vi "stage-controller.vi"() -> ()   [LabVIEW 2014]
uses:
  Stage SubVis/Move stage command - Global - SubVI.ctl
  Stage SubVis/user event out globals - SubVI.vi
  Stage SubVis/field-raster-globals.vi
  lib/Madlib/Madlib.lvlib
panel:
  in  "Current Z 2":ext(slide)=5.551115123125783e-17 scale=-1.0..1.0 scale format="%_1f"
  out "Current (X,Y)":cluster{ext[], ext[]}[](graph)=[{[101.064], [100.915]}, {[67.376, 134.75199999999998], [134.55333333333334, 134.55333333333334]}, {[67.376, 134.75199999999998], [67.27666666666667, 67.27666666666667]}]
  in  "Field Number":u32(slide)=1 min=1 max=16 step=1 scale=1.0..16.0
  in  "Field Size":enum16{"0", "1", "4", "9", "16"}(ring)=enum."9"
  in  "x-":bool
  in  "y+":bool
  in  "y-":bool
  in  "x+":bool
  out "Current Z (um)":ext
  out "Current X (um)":ext
  out "Current Y (um)":ext
  in  "Current Z":dbl(slide) min=0.0 step=0.5 scale=0.0..202.234 scale format="%#_4g"
  out "At limit 3":bool
  out "At limit 2":bool
  out "At limit":bool
  in  "x,y step (um)":ext=10.0 format="%_5g"
  in  "z step (um)":ext(slide)=0.1 scale=0.05..2.0 scale format="%#_2g"
  in  "z-":bool
  in  "z+":bool
  in  "Reset stage to center\n         (x, y, and z)":bool
  in  "STOP":bool
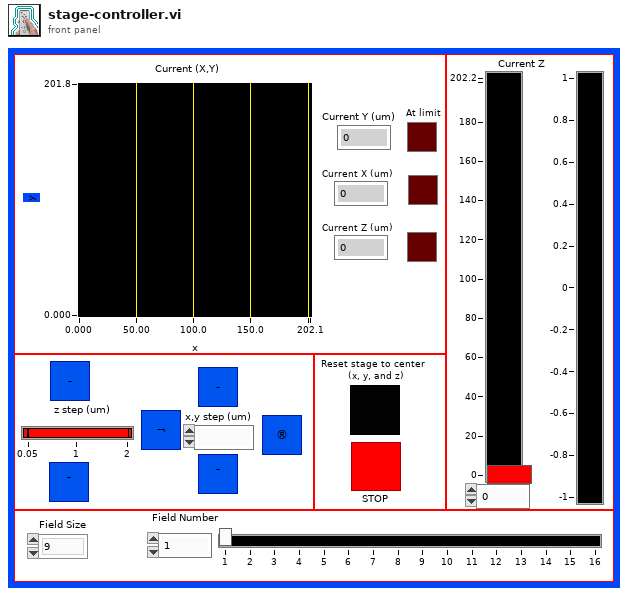
[diagram p1: front panel]
types:
  T1 = cluster{"X Command":dbl, "Y Command":dbl, "Z Command":dbl, "X Position":dbl, "Y Position":dbl, "Z Position":dbl, "X Calibration":dbl, "Y Calibration":dbl, "Z Calibration":dbl}
  T2 = typedef "Move stage command - Global - SubVI.ctl" = cluster{"dx (um) (0 -> ignore)":ext, "dy (um) (0 -> ignore)":ext, "dz (um) (0 -> ignore)":ext, "Re-center x,y":bool, "Re-center z":bool, "x (um) (-1 -> ignore)":dbl, "y (um) (-1 -> ignore)":dbl, "z (um) (-1 -> ignore)":dbl}
  T3 = typedef "small z increment.ctl" = dbl
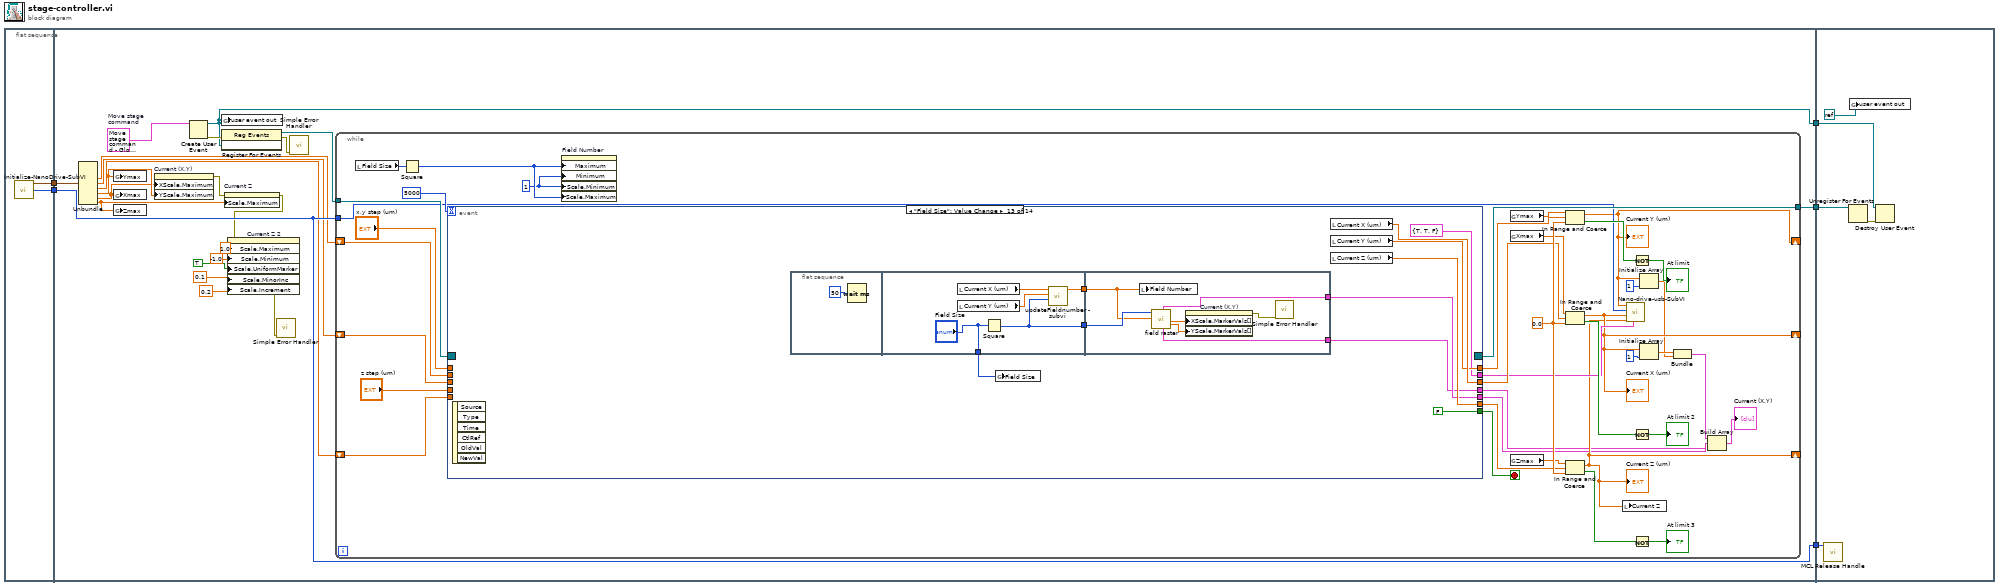
[diagram p0: block diagram]
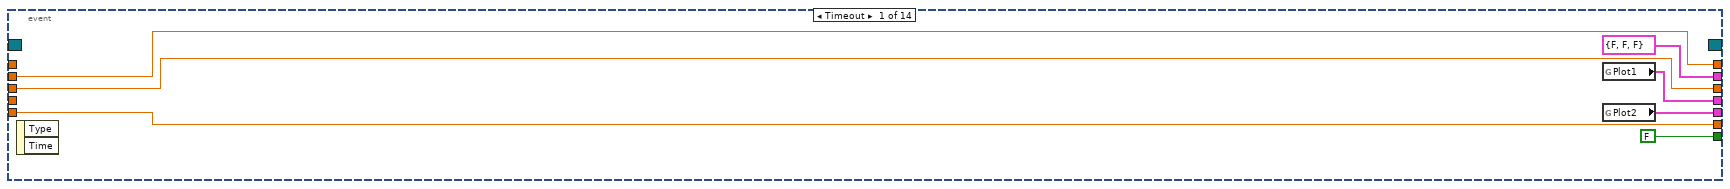
[diagram p2: hidden frame]
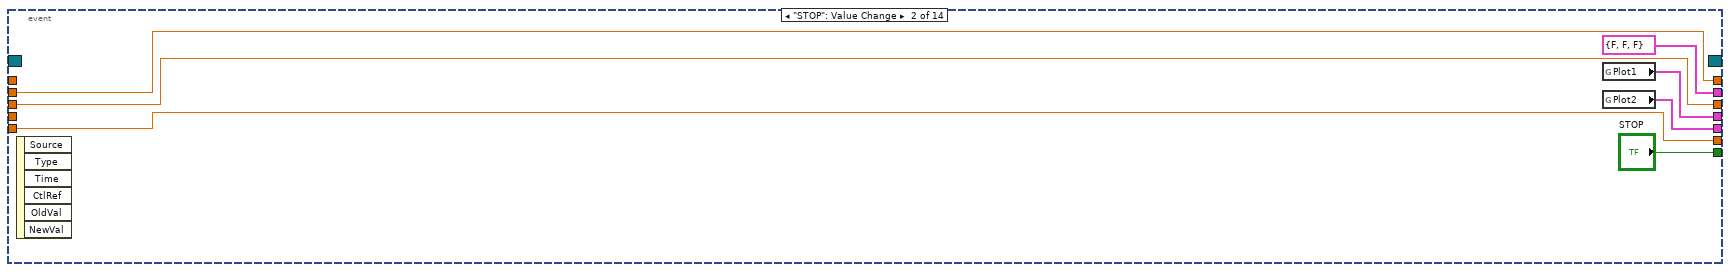
[diagram p3: hidden frame]
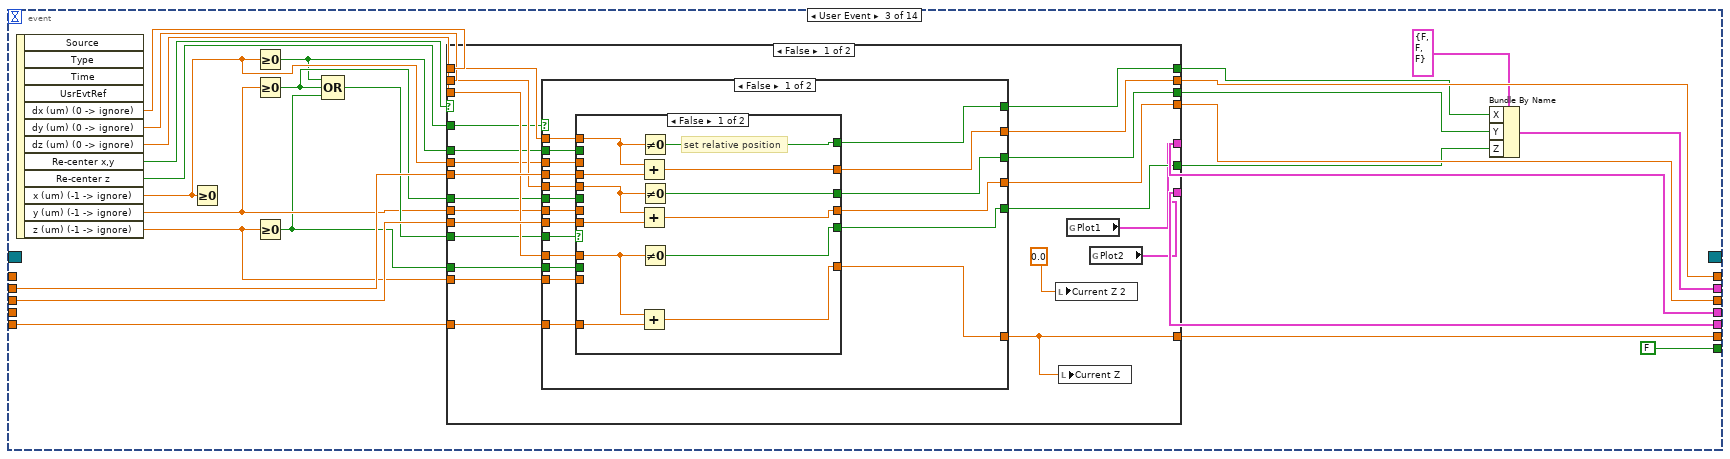
[diagram p4: hidden frame]
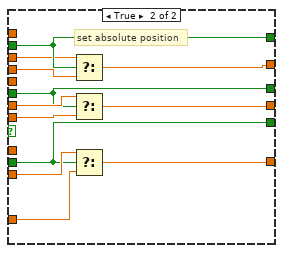
[diagram p5: hidden frame]
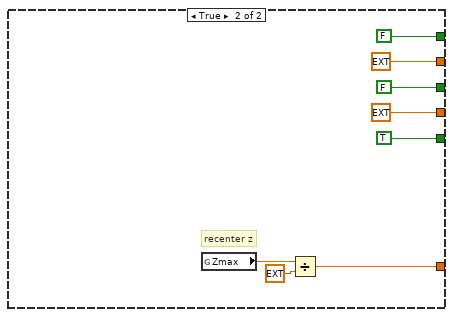
[diagram p6: hidden frame]
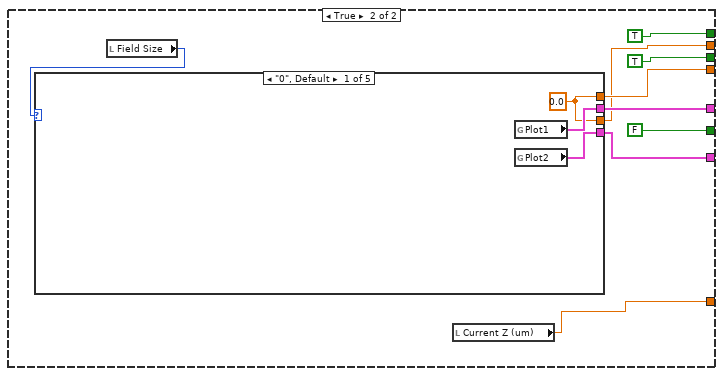
[diagram p7: hidden frame]
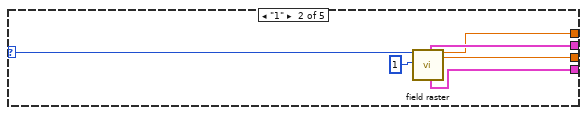
[diagram p8: hidden frame]
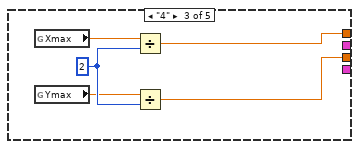
[diagram p9: hidden frame]
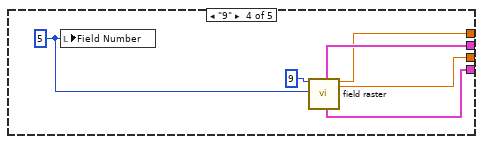
[diagram p10: hidden frame]
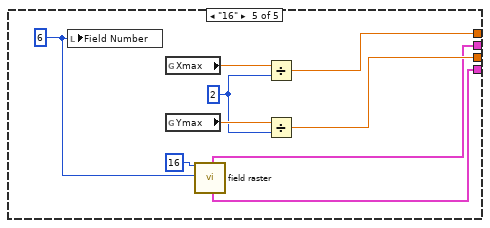
[diagram p11: hidden frame]
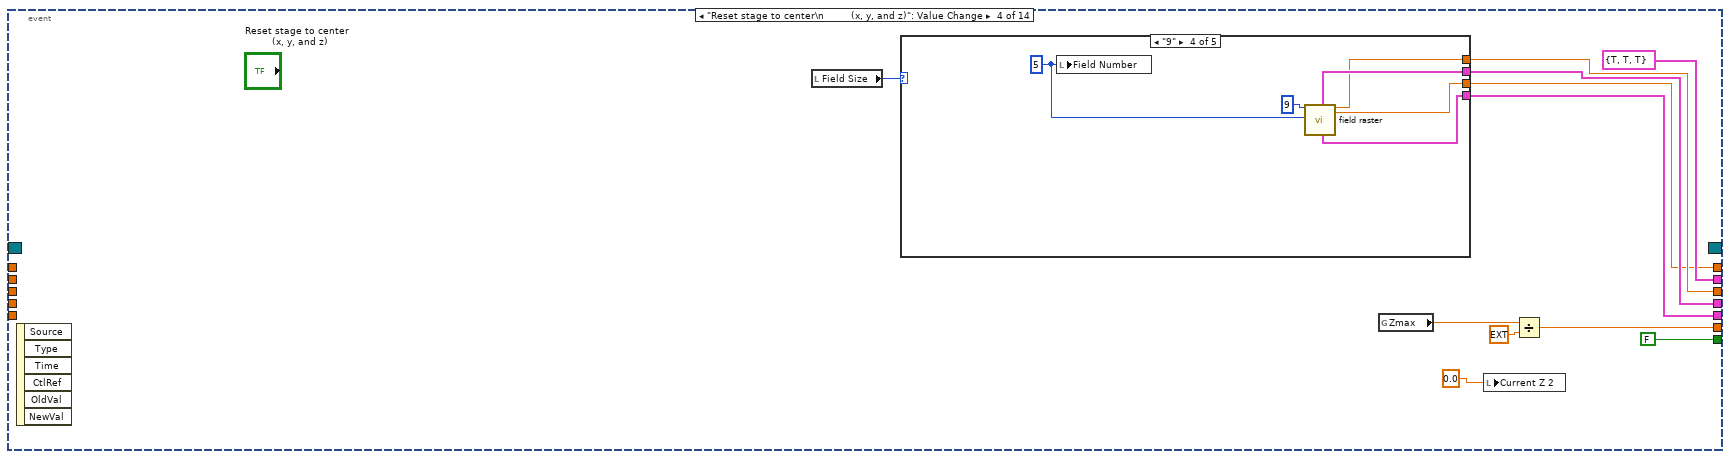
[diagram p12: hidden frame]
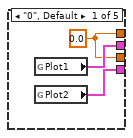
[diagram p13: hidden frame]
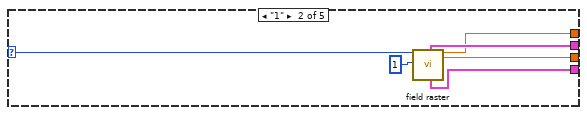
[diagram p14: hidden frame]
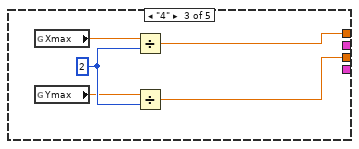
[diagram p15: hidden frame]
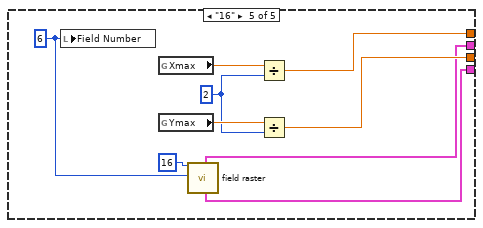
[diagram p16: hidden frame]
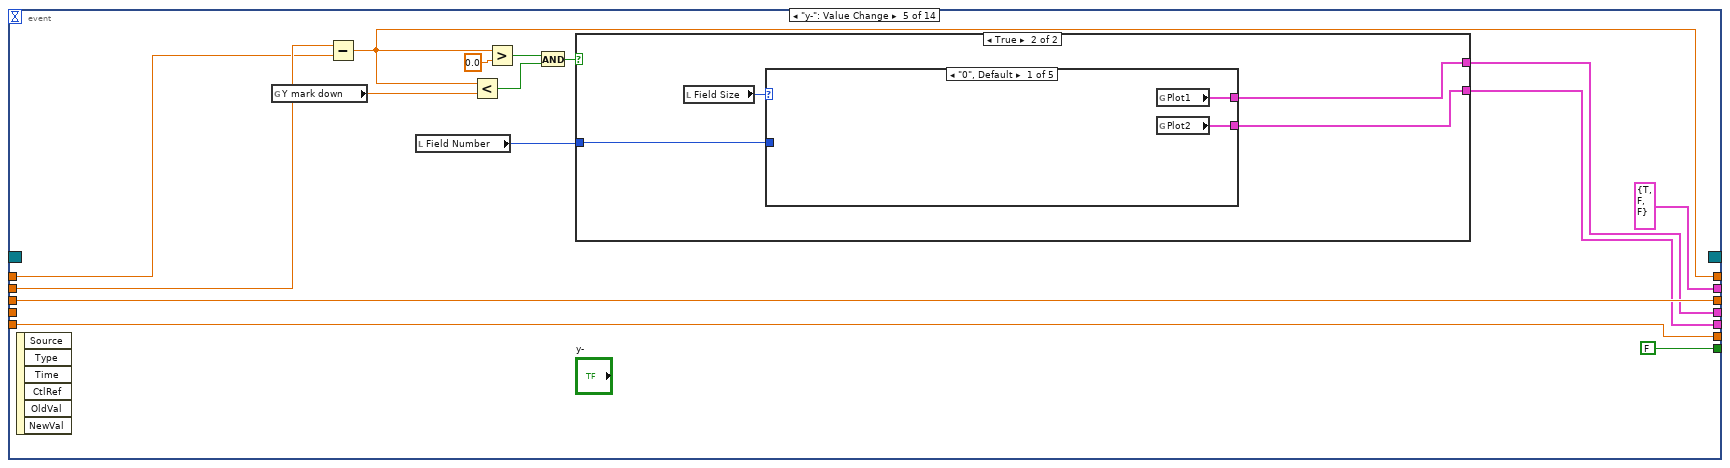
[diagram p17: hidden frame]
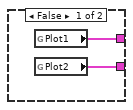
[diagram p18: hidden frame]
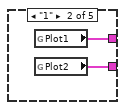
[diagram p19: hidden frame]
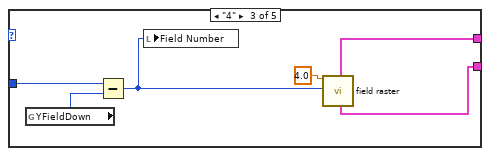
[diagram p20: hidden frame]
diagram:
  n1 = flat-sequence {
    tunnel: [w7] -> w5
    tunnel: [w6] -> w2
    tunnel: w5 -> [w29]
    tunnel: [w24] -> w4
    tunnel: [w23] -> w3
    tunnel: w2 -> [w22]
    tunnel: [w22] -> w1
    tunnel: w4 -> [w518]
    tunnel: w3 -> [w517]
    tunnel: w1 -> [w515]
    frame #0 {
      n2 = call "Initialize-NanoDrive-SubVI.vi"() -> ("Output Pos Info"=w7:T1, "Handle"=w6:i32)  [unwired: 1 in, 1 out]
    }
    frame #1 {
      w28 = T2 {"dx (um) (0 -> ignore)"=0.0, "dy (um) (0 -> ignore)"=0.0, "dz (um) (0 -> ignore)"=0.0, "Re-center x,y"=FALSE, "Re-center z"=FALSE, "x (um) (-1 -> ignore)"=-1.0, "y (um) (-1 -> ignore)"=-1.0, "z (um) (-1 -> ignore)"=-1.0}  # Move stage command
      n3 = Unbundle(w29) -> ("X Position"=w21:dbl, "Y Position"=w20:dbl, "Z Position"=w19:dbl, "X Calibration"=w17:dbl, "Y Calibration"=w16:dbl, "Z Calibration"=w15:dbl)  [unwired: 3 out]
      n4 = global write "field-raster-globals.vi" "Ymax"(w17) -> ()
      n5 = global write "field-raster-globals.vi" "Xmax"(w16) -> ()
      n6 = global write "field-raster-globals.vi" "Zmax"(w15) -> ()
      n7 = property on="Current (X,Y)" class="XYGraph (strict)"("XScale.Maximum"=w16, "YScale.Maximum"=w17) -> (error out=w18:errorcluster)  [unwired: 2 in, 1 out]
      n8 = Create User Event(user event datatype=w28) -> (user event=w23:refnum<user-event>, error out=w26:errorcluster)  [unwired: 1 in]
      n9 = global write "user event out globals - SubVI.vi" "user event out"(w23) -> ()
      n10 = register-events(error in=w26, w23) -> (reference out=w25:refnum<event-registration>, error out=w27:errorcluster)  [unwired: 1 in]
      n11 = property on="Current Z" class="Slide (strict)"(error in=w18, "Scale.Maximum"=w15) -> (error out=w14:errorcluster)  [unwired: 1 in, 1 out]
      n12 = property on="Current Z 2" class="Slide (strict)"(error in=w14, "Scale.Maximum"=1.0 ("Scale.Range:Maximum"), "Scale.Minimum"=-1.0 ("Scale.Range:Minimum"), "Scale.UniformMarker"=TRUE, "Scale.MinorInc"=0.1 ("Scale.Range:Minor Increment"), "Scale.Increment"=0.2 ("Scale.Range:Increment")) -> (error out=w13:errorcluster)  [unwired: 1 in, 1 out]
      n13 = call <vilib>:"Simple Error Handler.vi"("error in (no error)"=w13) -> ()  [unwired: 4 in, 5 out]
      n14 = call <vilib>:"Simple Error Handler.vi"("error in (no error)"=w27) -> ()  [unwired: 1 in, 8 out]
      n15 = while {
        tunnel: w25 -> [w65]
        tunnel: [w64] -> w24
        tunnel: w22 -> [w49]
        shift-right: [w45] -> _
        shift-left: w21 -> [w48]
        shift-right: [w44] -> _
        shift-left: w20 -> [w47]
        shift-right: [w40] -> _
        shift-left: w19 -> [w46]
        stop <- w66 stop-if-true
        w37 = 1
        w63 = 0.0
        n16 = local read "Field Size"() -> (w39:enum16{"0", "1", "4", "9", "16"})
        n17 = Square(x=w39) -> (x^2=w38:u16)
        n18 = event shown="[12] \"Field Size\": Value Change" {
          selector: w65 -> [_ _ _ _ _ _ _ _ _ _ _ _ _ _]
          dyn-events: [_ _ _ _ _ _ _ _ _ _ _ _ _ _] -> w64
          timeout: 5000 -> [_ _ _ _ _ _ _ _ _ _ _ _ _ _]
          tunnel: [FALSE ("Stop") "STOP" FALSE ("Stop") FALSE ("Stop") FALSE ("Stop") FALSE ("Stop") FALSE ("Stop") FALSE ("Stop") FALSE ("Stop") FALSE ("Stop") FALSE ("Stop") FALSE ("Stop") FALSE FALSE] -> w66
          tunnel: w48 -> [w73 w80 w107 _ w270 w310 w317 w328 w347 w358 w405 w445 _ _]
          tunnel: w47 -> [w72 w79 w106 _ w273 w305 w316 w327 w346 w362 w402 w449 _ _]
          tunnel: w46 -> [w71 w78 w105 _ w272 w307 _ w325 w343 w363 w406 w448 _ _]
          tunnel: [w73 w80 w102 w222 w261 w310 w317 w328 w347 w358 w405 w437 w487 w508] -> w62
          tunnel: [w72 w79 w103 w223 w273 w305 w316 w327 w346 w351 w394 w449 w488 w507] -> w61
          tunnel: [w71 w78 w104 w228 w272 w309 "Current Z" w324 w349 w363 w406 w448 w485 w503] -> w60
          tunnel: [cluster{"X":bool, "Y":bool, "Z":bool} {"X"=FALSE, "Y"=FALSE, "Z"=FALSE} ("Set this axis?") cluster{"X":bool, "Y":bool, "Z":bool} {"X"=FALSE, "Y"=FALSE, "Z"=FALSE} ("Set this axis?") w95 cluster{"X":bool, "Y":bool, "Z":bool} {"X"=TRUE, "Y"=TRUE, "Z"=TRUE} ("Set this axis?") cluster{"X":bool, "Y":bool, "Z":bool} {"X"=TRUE, "Y"=FALSE, "Z"=FALSE} ("Set this axis?") cluster{"X":bool, "Y":bool, "Z":bool} {"X"=FALSE, "Y"=FALSE, "Z"=TRUE} ("Set this axis?") cluster{"X":bool, "Y":bool, "Z":bool} {"X"=FALSE, "Y"=FALSE, "Z"=TRUE} ("Set this axis?") cluster{"X":bool, "Y":bool, "Z":bool} {"X"=FALSE, "Y"=FALSE, "Z"=TRUE} ("Set this axis?") cluster{"X":bool, "Y":bool, "Z":bool} {"X"=FALSE, "Y"=FALSE, "Z"=TRUE} ("Set this axis?") cluster{"X":bool, "Y":bool, "Z":bool} {"X"=FALSE, "Y"=TRUE, "Z"=FALSE} ("Set this axis?") cluster{"X":bool, "Y":bool, "Z":bool} {"X"=FALSE, "Y"=TRUE, "Z"=FALSE} ("Set this axis?") cluster{"X":bool, "Y":bool, "Z":bool} {"X"=TRUE, "Y"=FALSE, "Z"=FALSE} ("Set this axis?") cluster{"X":bool, "Y":bool, "Z":bool} {"X"=TRUE, "Y"=TRUE, "Z"=FALSE} ("Set this axis?") cluster{"X":bool, "Y":bool, "Z":bool} {"X"=TRUE, "Y"=TRUE, "Z"=FALSE} ("Set this axis?")] -> w50
          tunnel: "x,y step (um)" -> [_ _ _ _ w269 _ _ _ _ w361 w403 w446 _ _]
          tunnel: "z step (um)" -> [_ _ _ _ _ w306 _ _ w344 _ _ _ _ _]
          tunnel: [w68 w75 w82 w225 w266 w304 w313 w331 w342 w356 w399 w442 w483 w509] -> w35
          tunnel: [w69 w76 w83 w226 w267 w303 w314 w330 w341 w357 w400 w443 w482 w510] -> w34
          event Timeout {
            n19 = event-data() -> ()  [unwired: 3 out]
            n20 = global read "field-raster-globals.vi" "Plot1"() -> (w69:cluster{dbl[], dbl[]})
            n21 = global read "field-raster-globals.vi" "Plot2"() -> (w68:cluster{dbl[], dbl[]})
          }
          event "STOP": Value Change {
            n22 = event-data() -> ()  [unwired: 7 out]
            n23 = global read "field-raster-globals.vi" "Plot1"() -> (w76:cluster{dbl[], dbl[]})
            n24 = global read "field-raster-globals.vi" "Plot2"() -> (w75:cluster{dbl[], dbl[]})
          }
          event User Event {
            n25 = event-data() -> ("dx (um) (0 -> ignore)"=w100:ext, "dy (um) (0 -> ignore)"=w99:ext, "dz (um) (0 -> ignore)"=w98:ext, "Re-center x,y"=w97:bool, "Re-center z"=w91:bool, "x (um) (-1 -> ignore)"=w87:dbl, "y (um) (-1 -> ignore)"=w88:dbl, "z (um) (-1 -> ignore)"=w89:dbl)  [unwired: 5 out]
            n26 = Greater Or Equal To 0?(x=w87) -> ()  [unwired: 1 out]
            n27 = Greater Or Equal To 0?(x=w87) -> (x >= 0?=w84:bool)
            n28 = Greater Or Equal To 0?(x=w88) -> (x >= 0?=w85:bool)
            n29 = Greater Or Equal To 0?(x=w89) -> (x >= 0?=w86:bool)
            n30 = Compound Arithmetic op=OR(w84, w85, w86) -> (w90:bool)
            n31 = case shown="False" w97 {
              tunnel: w107 -> [w130 _]
              tunnel: w106 -> [w129 _]
              tunnel: w105 -> [w128 _]
              tunnel: [w111 w183] -> w104
              tunnel: [w127 w185] -> w103
              tunnel: [w126 w184] -> w102
              tunnel: w100 -> [w125 _]
              tunnel: w99 -> [w124 _]
              tunnel: w98 -> [w123 _]
              tunnel: [w122 FALSE] -> w94
              tunnel: [w121 TRUE] -> w93
              tunnel: [w120 TRUE] -> w92
              tunnel: w91 -> [w119 _]
              tunnel: w90 -> [w118 _]
              tunnel: w89 -> [w117 _]
              tunnel: w88 -> [w116 _]
              tunnel: w87 -> [w115 _]
              tunnel: w86 -> [w114 _]
              tunnel: w85 -> [w113 _]
              tunnel: w84 -> [w112 _]
              tunnel: [w109 w187] -> w83
              tunnel: [w108 w186] -> w82
              frame False {
                n32 = case shown="False" w119 {
                  tunnel: w130 -> [w149 _]
                  tunnel: w129 -> [w148 _]
                  tunnel: w128 -> [w147 _]
                  tunnel: [w146 w180] -> w111
                  tunnel: [w145 ext 0.0] -> w127
                  tunnel: [w144 ext 0.0] -> w126
                  tunnel: w125 -> [w143 _]
                  tunnel: w124 -> [w142 _]
                  tunnel: w123 -> [w141 _]
                  tunnel: [w140 TRUE] -> w122
                  tunnel: [w139 FALSE] -> w121
                  tunnel: [w138 FALSE] -> w120
                  tunnel: w118 -> [w137 _]
                  tunnel: w117 -> [w136 _]
                  tunnel: w116 -> [w135 _]
                  tunnel: w115 -> [w134 _]
                  tunnel: w114 -> [w133 _]
                  tunnel: w113 -> [w132 _]
                  tunnel: w112 -> [w131 _]
                  frame False {
                    n33 = case shown="False" w137 {
                      tunnel: w149 -> [w161 w169]
                      tunnel: w148 -> [w160 w166]
                      tunnel: w147 -> [w159 w163]
                      tunnel: [w158 w165] -> w146
                      tunnel: [w157 w168] -> w145
                      tunnel: [w156 w172] -> w144
                      tunnel: w143 -> [w155 _]
                      tunnel: w142 -> [w154 _]
                      tunnel: w141 -> [w153 _]
                      tunnel: [w152 w162] -> w140
                      tunnel: [w151 w167] -> w139
                      tunnel: [w150 w171] -> w138
                      tunnel: w136 -> [_ w164]
                      tunnel: w135 -> [_ w173]
                      tunnel: w134 -> [_ w170]
                      tunnel: w133 -> [_ w162]
                      tunnel: w132 -> [_ w167]
                      tunnel: w131 -> [_ w171]
                      frame False {
                        # "set relative position"
                        n34 = Add(x=w155, y=w161) -> (x+y=w156:ext)
                        n35 = Add(x=w154, y=w160) -> (x+y=w157:ext)
                        n36 = Add(x=w153, y=w159) -> (x+y=w158:ext)
                        n37 = Not Equal To 0?(x=w155) -> (x != 0?=w150:bool)
                        n38 = Not Equal To 0?(x=w154) -> (x != 0?=w151:bool)
                        n39 = Not Equal To 0?(x=w153) -> (x != 0?=w152:bool)
                      }
                      frame True {
                        # "set absolute position"
                        n40 = Select(t=w170, s=w171, f=w169) -> (s? t:f=w172:ext)
                        n41 = Select(t=w173, s=w167, f=w166) -> (s? t:f=w168:ext)
                        n42 = Select(t=w164, s=w162, f=w163) -> (s? t:f=w165:ext)
                      }
                    }
                  }
                  frame True {
                    # "recenter z"
                    n43 = global read "field-raster-globals.vi" "Zmax"() -> (w174:dbl)
                    n44 = Divide(x=w174, y=ext 2.0) -> (x/y=w180:ext)
                  }
                }
                n45 = local write "Current Z 2"(0.0) -> ()
                n46 = local write "Current Z"(w111) -> ()
                n47 = global read "field-raster-globals.vi" "Plot1"() -> (w109:cluster{dbl[], dbl[]})
                n48 = global read "field-raster-globals.vi" "Plot2"() -> (w108:cluster{dbl[], dbl[]})
              }
              frame True {
                n49 = local read "Field Size"() -> (w182:enum16{"0", "1", "4", "9", "16"})
                n50 = case shown="\"0\", Default" w182 {
                  selector: w182 -> [_ w197 _ _ _]
                  tunnel: [w192 w199 _ w208 w214] -> w187
                  tunnel: [w193 w198 _ w207 w213] -> w186
                  tunnel: [w191 w195 w204 w206 w217] -> w184
                  tunnel: [w191 w194 w203 w205 w216] -> w185
                  frame "0", Default {
                    w191 = 0.0
                    n51 = global read "field-raster-globals.vi" "Plot1"() -> (w192:cluster{dbl[], dbl[]})
                    n52 = global read "field-raster-globals.vi" "Plot2"() -> (w193:cluster{dbl[], dbl[]})
                  }
                  frame "1" {
                    n53 = call "field raster.vi"("field size"=w197, "field number"=1) -> ("Plot1"=w199:cluster{dbl[], dbl[]}, "Plot2"=w198:cluster{dbl[], dbl[]}, "current X"=w194:dbl, "current Y"=w195:dbl)  [unwired: 12 in, 2 out]
                  }
                  frame "4" {
                    w202 = 2
                    n54 = global read "field-raster-globals.vi" "Xmax"() -> (w201:dbl)
                    n55 = global read "field-raster-globals.vi" "Ymax"() -> (w200:dbl)
                    n56 = Divide(x=w201, y=w202) -> (x/y=w203:dbl)
                    n57 = Divide(x=w200, y=w202) -> (x/y=w204:dbl)
                  }
                  frame "9" {
                    w209 = 5
                    n58 = local write "Field Number"(w209) -> ()
                    n59 = call "field raster.vi"("field size"=9, "field number"=w209) -> ("Plot1"=w208:cluster{dbl[], dbl[]}, "Plot2"=w207:cluster{dbl[], dbl[]}, "current X"=w205:dbl, "current Y"=w206:dbl)  [unwired: 12 in, 2 out]
                  }
                  frame "16" {
                    w212 = 2
                    w211 = 6
                    n60 = local write "Field Number"(w211) -> ()
                    n61 = global read "field-raster-globals.vi" "Xmax"() -> (w218:dbl)
                    n62 = global read "field-raster-globals.vi" "Ymax"() -> (w219:dbl)
                    n63 = call "field raster.vi"("field size"=16, "field number"=w211) -> ("Plot1"=w214:cluster{dbl[], dbl[]}, "Plot2"=w213:cluster{dbl[], dbl[]})  [unwired: 12 in, 4 out]
                    n64 = Divide(x=w218, y=w212) -> (x/y=w216:dbl)
                    n65 = Divide(x=w219, y=w212) -> (x/y=w217:dbl)
                  }
                }
                n66 = local read "Current Z (um)"() -> (w183:ext)
              }
            }
            n67 = Bundle By Name(cluster=cluster{"X":bool, "Y":bool, "Z":bool} {"X"=FALSE, "Y"=FALSE, "Z"=FALSE} ("Set this axis?"), "X"=w92, "Y"=w93, "Z"=w94) -> (w95:cluster{"X":bool, "Y":bool, "Z":bool})
          }
          event "Reset stage to center\n         (x, y, and z)": Value Change {
            n68 = event-data() -> ()  [unwired: 7 out]
            n69 = local read "Field Size"() -> (w224:enum16{"0", "1", "4", "9", "16"})
            n70 = case shown="\"9\"" w224 {
              selector: w224 -> [_ w237 _ _ _]
              tunnel: [w232 w239 _ w248 w254] -> w226
              tunnel: [w233 w238 _ w247 w253] -> w225
              tunnel: [w231 w235 w244 w246 w257] -> w222
              tunnel: [w231 w234 w243 w245 w256] -> w223
              frame "0", Default {
                w231 = 0.0
                n71 = global read "field-raster-globals.vi" "Plot1"() -> (w232:cluster{dbl[], dbl[]})
                n72 = global read "field-raster-globals.vi" "Plot2"() -> (w233:cluster{dbl[], dbl[]})
              }
              frame "1" {
                n73 = call "field raster.vi"("field size"=w237, "field number"=1) -> ("Plot1"=w239:cluster{dbl[], dbl[]}, "Plot2"=w238:cluster{dbl[], dbl[]}, "current X"=w234:dbl, "current Y"=w235:dbl)  [unwired: 12 in, 2 out]
              }
              frame "4" {
                w242 = 2
                n74 = global read "field-raster-globals.vi" "Xmax"() -> (w241:dbl)
                n75 = global read "field-raster-globals.vi" "Ymax"() -> (w240:dbl)
                n76 = Divide(x=w241, y=w242) -> (x/y=w243:dbl)
                n77 = Divide(x=w240, y=w242) -> (x/y=w244:dbl)
              }
              frame "9" {
                w249 = 5
                n78 = local write "Field Number"(w249) -> ()
                n79 = call "field raster.vi"("field size"=9, "field number"=w249) -> ("Plot1"=w248:cluster{dbl[], dbl[]}, "Plot2"=w247:cluster{dbl[], dbl[]}, "current X"=w245:dbl, "current Y"=w246:dbl)  [unwired: 12 in, 2 out]
              }
              frame "16" {
                w252 = 2
                w251 = 6
                n80 = local write "Field Number"(w251) -> ()
                n81 = global read "field-raster-globals.vi" "Xmax"() -> (w258:dbl)
                n82 = global read "field-raster-globals.vi" "Ymax"() -> (w259:dbl)
                n83 = call "field raster.vi"("field size"=16, "field number"=w251) -> ("Plot1"=w254:cluster{dbl[], dbl[]}, "Plot2"=w253:cluster{dbl[], dbl[]})  [unwired: 12 in, 4 out]
                n84 = Divide(x=w258, y=w252) -> (x/y=w256:dbl)
                n85 = Divide(x=w259, y=w252) -> (x/y=w257:dbl)
              }
            }
            n86 = global read "field-raster-globals.vi" "Zmax"() -> (w221:dbl)
            n87 = local write "Current Z 2"(0.0) -> ()
            n88 = Divide(x=w221, y=ext 2.0) -> (x/y=w228:ext)
          }
          event "y-": Value Change {
            n89 = event-data() -> ()  [unwired: 7 out]
            n90 = global read "field-raster-globals.vi" "Y mark down"() -> (w268:dbl)
            n91 = Subtract(x=w270, y=w269) -> (x-y=w261:ext)
            n92 = local read "Field Number"() -> (w260:u32)
            n93 = Less?(x=w261, y=w268) -> (x < y?=w265:bool)
            n94 = Greater?(x=w261, y=0.0) -> (0:w263:bool)
            n95 = And(x=w263, y=w265) -> (x .and. y?=w264:bool)
            n96 = case shown="True" w264 {
              tunnel: [w276 w279] -> w267
              tunnel: [w275 w278] -> w266
              tunnel: w260 -> [_ w277]
              frame False {
                n97 = global read "field-raster-globals.vi" "Plot1"() -> (w276:cluster{dbl[], dbl[]})
                n98 = global read "field-raster-globals.vi" "Plot2"() -> (w275:cluster{dbl[], dbl[]})
              }
              frame True {
                n99 = local read "Field Size"() -> (w280:enum16{"0", "1", "4", "9", "16"})
                n100 = case shown="\"0\", Default" w280 {
                  tunnel: w277 -> [_ _ w286 w296 w301]
                  tunnel: [w282 w284 w289 w294 w299] -> w279
                  tunnel: [w281 w283 w290 w293 w298] -> w278
                  frame "0", Default {
                    n101 = global read "field-raster-globals.vi" "Plot1"() -> (w282:cluster{dbl[], dbl[]})
                    n102 = global read "field-raster-globals.vi" "Plot2"() -> (w281:cluster{dbl[], dbl[]})
                  }
                  frame "1" {
                    n103 = global read "field-raster-globals.vi" "Plot1"() -> (w284:cluster{dbl[], dbl[]})
                    n104 = global read "field-raster-globals.vi" "Plot2"() -> (w283:cluster{dbl[], dbl[]})
                  }
                  frame "4" {
                    n105 = global read "field-raster-globals.vi" "YFieldDown"() -> (w285:u32)
                    n106 = Subtract(x=w286, y=w285) -> (x-y=w287:u32)
                    n107 = local write "Field Number"(w287) -> ()
                    n108 = call "field raster.vi"("field size"=4.0, "field number"=w287) -> ("Plot1"=w289:cluster{dbl[], dbl[]}, "Plot2"=w290:cluster{dbl[], dbl[]})  [unwired: 12 in, 4 out]
                  }
                  frame "9" {
                    n109 = global read "field-raster-globals.vi" "YFieldDown"() -> (w292:u32)
                    n110 = Subtract(x=w296, y=w292) -> (x-y=w291:u32)
                    n111 = local write "Field Number"(w291) -> ()
                    n112 = call "field raster.vi"("field size"=9, "field number"=w291) -> ("Plot1"=w294:cluster{dbl[], dbl[]}, "Plot2"=w293:cluster{dbl[], dbl[]})  [unwired: 12 in, 4 out]
                  }
                  frame "16" {
                    n113 = global read "field-raster-globals.vi" "YFieldDown"() -> (w297:u32)
                    n114 = Subtract(x=w301, y=w297) -> (x-y=w300:u32)
                    n115 = local write "Field Number"(w300) -> ()
                    n116 = call "field raster.vi"("field size"=16, "field number"=w300) -> ("Plot1"=w299:cluster{dbl[], dbl[]}, "Plot2"=w298:cluster{dbl[], dbl[]})  [unwired: 12 in, 4 out]
                  }
                }
              }
            }
          }
          event "z+": Value Change {
            n117 = event-data() -> ()  [unwired: 7 out]
            n118 = Add(x=w306, y=w307) -> (x+y=w309:ext)
            n119 = global read "field-raster-globals.vi" "Plot1"() -> (w303:cluster{dbl[], dbl[]})
            n120 = global read "field-raster-globals.vi" "Plot2"() -> (w304:cluster{dbl[], dbl[]})
          }
          event "Current Z": Mouse Up {
            w312 = 0.0
            n121 = event-data() -> ()  [unwired: 5 out]
            n122 = global write "field-raster-globals.vi" "Previous small Z increment"(w312) -> ()
            n123 = local write "Current Z 2"(w312) -> ()
            n124 = global read "field-raster-globals.vi" "Plot1"() -> (w314:cluster{dbl[], dbl[]})
            n125 = global read "field-raster-globals.vi" "Plot2"() -> (w313:cluster{dbl[], dbl[]})
          }
          event "Current Z 2": Mouse Up {
            n126 = event-data() -> ()  [unwired: 8 out]
            n127 = global read "field-raster-globals.vi" "Previous small Z increment"() -> (w323:T3)
            n128 = Subtract(x="Current Z 2", y=w323) -> (x-y=w321:ext)
            n129 = Greater?(x=w321, y=0.0) -> (0:w326:bool)
            n130 = case shown="True" w326 {
              tunnel: w325 -> [w333 w339]
              tunnel: w321 -> [w334 w338]
              tunnel: [w336 w340] -> w324
              tunnel: "Current Z 2" -> [w335 w337]
              frame False {
                n131 = global write "field-raster-globals.vi" "Previous small Z increment"(w335) -> ()
                n132 = Add(x=w333, y=w334) -> (x+y=w336:ext)
              }
              frame True {
                n133 = global write "field-raster-globals.vi" "Previous small Z increment"(w337) -> ()
                n134 = Add(x=w339, y=w338) -> (x+y=w340:ext)
              }
            }
            n135 = global read "field-raster-globals.vi" "Plot1"() -> (w330:cluster{dbl[], dbl[]})
            n136 = global read "field-raster-globals.vi" "Plot2"() -> (w331:cluster{dbl[], dbl[]})
          }
          event "z-": Value Change {
            n137 = event-data() -> ()  [unwired: 7 out]
            n138 = Subtract(x=w343, y=w344) -> (x-y=w349:ext)
            n139 = global read "field-raster-globals.vi" "Plot1"() -> (w341:cluster{dbl[], dbl[]})
            n140 = global read "field-raster-globals.vi" "Plot2"() -> (w342:cluster{dbl[], dbl[]})
          }
          event "x+": Value Change {
            n141 = event-data() -> ()  [unwired: 7 out]
            n142 = Add(x=w361, y=w362) -> (x+y=w351:ext)
            n143 = global read "field-raster-globals.vi" "X mark up"() -> (w359:dbl)
            n144 = global read "field-raster-globals.vi" "Xmax"() -> (w352:dbl)
            n145 = local read "Field Number"() -> (w350:u32)
            n146 = Less?(x=w351, y=w352) -> (x < y?=w353:bool)
            n147 = Greater?(x=w351, y=w359) -> (0:w354:bool)
            n148 = And(x=w353, y=w354) -> (x .and. y?=w355:bool)
            n149 = case shown="True" w355 {
              tunnel: [w366 w369] -> w357
              tunnel: [w365 w368] -> w356
              tunnel: w350 -> [_ w367]
              frame False {
                n150 = global read "field-raster-globals.vi" "Plot1"() -> (w366:cluster{dbl[], dbl[]})
                n151 = global read "field-raster-globals.vi" "Plot2"() -> (w365:cluster{dbl[], dbl[]})
              }
              frame True {
                n152 = local read "Field Size"() -> (w370:enum16{"0", "1", "4", "9", "16"})
                n153 = case shown="\"4\"" w370 {
                  tunnel: w367 -> [_ _ w376 w386 w391]
                  tunnel: [w372 w374 w379 w384 w389] -> w369
                  tunnel: [w371 w373 w380 w383 w388] -> w368
                  frame "0", Default {
                    n154 = global read "field-raster-globals.vi" "Plot1"() -> (w372:cluster{dbl[], dbl[]})
                    n155 = global read "field-raster-globals.vi" "Plot2"() -> (w371:cluster{dbl[], dbl[]})
                  }
                  frame "1" {
                    n156 = global read "field-raster-globals.vi" "Plot1"() -> (w374:cluster{dbl[], dbl[]})
                    n157 = global read "field-raster-globals.vi" "Plot1"() -> (w373:cluster{dbl[], dbl[]})
                  }
                  frame "4" {
                    n158 = global read "field-raster-globals.vi" "XFieldDiff"() -> (w375:dbl)
                    n159 = Add(x=w376, y=w375) -> (x+y=w377:dbl)
                    n160 = local write "Field Number"(w377) -> ()
                    n161 = call "field raster.vi"("field size"=4.0, "field number"=w377) -> ("Plot1"=w379:cluster{dbl[], dbl[]}, "Plot2"=w380:cluster{dbl[], dbl[]})  [unwired: 12 in, 4 out]
                  }
                  frame "9" {
                    n162 = global read "field-raster-globals.vi" "XFieldDiff"() -> (w381:dbl)
                    n163 = Add(x=w386, y=w381) -> (x+y=w382:dbl)
                    n164 = local write "Field Number"(w382) -> ()
                    n165 = call "field raster.vi"("field size"=9, "field number"=w382) -> ("Plot1"=w384:cluster{dbl[], dbl[]}, "Plot2"=w383:cluster{dbl[], dbl[]})  [unwired: 12 in, 4 out]
                  }
                  frame "16" {
                    n166 = global read "field-raster-globals.vi" "XFieldDiff"() -> (w387:dbl)
                    n167 = Add(x=w391, y=w387) -> (x+y=w390:dbl)
                    n168 = local write "Field Number"(w390) -> ()
                    n169 = call "field raster.vi"("field size"=16, "field number"=w390) -> ("Plot1"=w389:cluster{dbl[], dbl[]}, "Plot2"=w388:cluster{dbl[], dbl[]})  [unwired: 12 in, 4 out]
                  }
                }
              }
            }
          }
          event "x-": Value Change {
            n170 = event-data() -> ()  [unwired: 7 out]
            n171 = global read "field-raster-globals.vi" "X mark down"() -> (w401:dbl)
            n172 = Subtract(x=w402, y=w403) -> (x-y=w394:ext)
            n173 = local read "Field Number"() -> (w393:u32)
            n174 = Less?(x=w394, y=w401) -> (x < y?=w397:bool)
            n175 = Greater?(x=w394, y=ext 0.0) -> (0:w396:bool)
            n176 = And(x=w396, y=w397) -> (x .and. y?=w398:bool)
            n177 = case shown="True" w398 {
              tunnel: [w409 w412] -> w400
              tunnel: [w408 w411] -> w399
              tunnel: w393 -> [_ w410]
              frame False {
                n178 = global read "field-raster-globals.vi" "Plot1"() -> (w409:cluster{dbl[], dbl[]})
                n179 = global read "field-raster-globals.vi" "Plot2"() -> (w408:cluster{dbl[], dbl[]})
              }
              frame True {
                n180 = local read "Field Size"() -> (w413:enum16{"0", "1", "4", "9", "16"})
                n181 = case shown="\"0\", Default" w413 {
                  tunnel: w410 -> [_ _ w419 w429 w434]
                  tunnel: [w415 w417 w422 w427 w432] -> w412
                  tunnel: [w414 w416 w423 w426 w431] -> w411
                  frame "0", Default {
                    n182 = global read "field-raster-globals.vi" "Plot1"() -> (w415:cluster{dbl[], dbl[]})
                    n183 = global read "field-raster-globals.vi" "Plot2"() -> (w414:cluster{dbl[], dbl[]})
                  }
                  frame "1" {
                    n184 = global read "field-raster-globals.vi" "Plot1"() -> (w417:cluster{dbl[], dbl[]})
                    n185 = global read "field-raster-globals.vi" "Plot2"() -> (w416:cluster{dbl[], dbl[]})
                  }
                  frame "4" {
                    n186 = global read "field-raster-globals.vi" "XFieldDiff"() -> (w418:dbl)
                    n187 = Subtract(x=w419, y=w418) -> (x-y=w420:dbl)
                    n188 = local write "Field Number"(w420) -> ()
                    n189 = call "field raster.vi"("field size"=4.0, "field number"=w420) -> ("Plot1"=w422:cluster{dbl[], dbl[]}, "Plot2"=w423:cluster{dbl[], dbl[]})  [unwired: 12 in, 4 out]
                  }
                  frame "9" {
                    n190 = global read "field-raster-globals.vi" "XFieldDiff"() -> (w424:dbl)
                    n191 = Subtract(x=w429, y=w424) -> (x-y=w425:dbl)
                    n192 = local write "Field Number"(w425) -> ()
                    n193 = call "field raster.vi"("field size"=9, "field number"=w425) -> ("Plot1"=w427:cluster{dbl[], dbl[]}, "Plot2"=w426:cluster{dbl[], dbl[]})  [unwired: 12 in, 4 out]
                  }
                  frame "16" {
                    n194 = global read "field-raster-globals.vi" "XFieldDiff"() -> (w430:dbl)
                    n195 = Subtract(x=w434, y=w430) -> (x-y=w433:dbl)
                    n196 = local write "Field Number"(w433) -> ()
                    n197 = call "field raster.vi"("field size"=16, "field number"=w433) -> ("Plot1"=w432:cluster{dbl[], dbl[]}, "Plot2"=w431:cluster{dbl[], dbl[]})  [unwired: 12 in, 4 out]
                  }
                }
              }
            }
          }
          event "y+": Value Change {
            n198 = event-data() -> ()  [unwired: 7 out]
            n199 = Add(x=w445, y=w446) -> (x+y=w437:ext)
            n200 = global read "field-raster-globals.vi" "Y mark up"() -> (w444:dbl)
            n201 = global read "field-raster-globals.vi" "Ymax"() -> (w438:dbl)
            n202 = local read "Field Number"() -> (w436:u32)
            n203 = Less?(x=w437, y=w438) -> (x < y?=w439:bool)
            n204 = Greater?(x=w437, y=w444) -> (0:w440:bool)
            n205 = And(x=w439, y=w440) -> (x .and. y?=w441:bool)
            n206 = case shown="True" w441 {
              tunnel: [w452 w455] -> w443
              tunnel: [w451 w454] -> w442
              tunnel: w436 -> [_ w453]
              frame False {
                n207 = global read "field-raster-globals.vi" "Plot1"() -> (w452:cluster{dbl[], dbl[]})
                n208 = global read "field-raster-globals.vi" "Plot2"() -> (w451:cluster{dbl[], dbl[]})
              }
              frame True {
                n209 = local read "Field Size"() -> (w456:enum16{"0", "1", "4", "9", "16"})
                n210 = case shown="\"1\"" w456 {
                  tunnel: w453 -> [_ _ w462 w472 w477]
                  tunnel: [w458 w460 w465 w470 w475] -> w455
                  tunnel: [w457 w459 w466 w469 w474] -> w454
                  frame "0", Default {
                    n211 = global read "field-raster-globals.vi" "Plot1"() -> (w458:cluster{dbl[], dbl[]})
                    n212 = global read "field-raster-globals.vi" "Plot2"() -> (w457:cluster{dbl[], dbl[]})
                  }
                  frame "1" {
                    n213 = global read "field-raster-globals.vi" "Plot1"() -> (w460:cluster{dbl[], dbl[]})
                    n214 = global read "field-raster-globals.vi" "Plot2"() -> (w459:cluster{dbl[], dbl[]})
                  }
                  frame "4" {
                    n215 = global read "field-raster-globals.vi" "YFieldUp"() -> (w461:u32)
                    n216 = Add(x=w462, y=w461) -> (x+y=w463:u32)
                    n217 = local write "Field Number"(w463) -> ()
                    n218 = call "field raster.vi"("field size"=4.0, "field number"=w463) -> ("Plot1"=w465:cluster{dbl[], dbl[]}, "Plot2"=w466:cluster{dbl[], dbl[]})  [unwired: 12 in, 4 out]
                  }
                  frame "9" {
                    n219 = global read "field-raster-globals.vi" "YFieldUp"() -> (w467:u32)
                    n220 = Add(x=w472, y=w467) -> (x+y=w468:u32)
                    n221 = local write "Field Number"(w468) -> ()
                    n222 = call "field raster.vi"("field size"=9, "field number"=w468) -> ("Plot1"=w470:cluster{dbl[], dbl[]}, "Plot2"=w469:cluster{dbl[], dbl[]})  [unwired: 12 in, 4 out]
                  }
                  frame "16" {
                    n223 = global read "field-raster-globals.vi" "YFieldUp"() -> (w473:u32)
                    n224 = Add(x=w477, y=w473) -> (x+y=w476:u32)
                    n225 = local write "Field Number"(w476) -> ()
                    n226 = call "field raster.vi"("field size"=16, "field number"=w476) -> ("Plot1"=w475:cluster{dbl[], dbl[]}, "Plot2"=w474:cluster{dbl[], dbl[]})  [unwired: 12 in, 4 out]
                  }
                }
              }
            }
          }
          event "Field Size": Value Change {
            n227 = event-data() -> ()  [unwired: 7 out]
            n228 = flat-sequence {
              tunnel: [w491] -> w481
              tunnel: [w494] -> w480
              tunnel: ["Field Size"] -> w479
              tunnel: [w501] -> w483
              tunnel: [w500] -> w482
              tunnel: w481 -> [w499]
              tunnel: w480 -> [w498]
              frame #0 {
                n229 = Wait (ms)(milliseconds to wait=50) -> ()  [unwired: 1 out]
              }
              frame #1 {
                n230 = local read "Current X (um)"() -> (w492:ext)
                n231 = local read "Current Y (um)"() -> (w493:ext)
                n232 = Square(x="Field Size") -> (x^2=w491:u16)
                n233 = call "updateFieldnumber - subvi.vi"("Field Size"=w491, "CurY"=w493, "CurX"=w492) -> ("Field Number"=w494:dbl)  [unwired: 8 in]
              }
              frame #2 {
                n234 = local write "Field Number"(w498) -> ()
                n235 = call "field raster.vi"("field size"=w499, "field number"=w498) -> ("Plot1"=w501:cluster{dbl[], dbl[]}, "Plot2"=w500:cluster{dbl[], dbl[]}, "x mark"=w496:dbl[], "y mark"=w495:dbl[])  [unwired: 12 in, 2 out]
                n236 = property on="Current (X,Y)" class="XYGraph (strict)"("XScale.MarkerVals[]"=w496, "YScale.MarkerVals[]"=w495) -> (error out=w497:errorcluster)  [unwired: 2 in, 1 out]
                n237 = call <vilib>:"Simple Error Handler.vi"("error in (no error)"=w497) -> ()  [unwired: 4 in, 5 out]
              }
            }
            n238 = global write "field-raster-globals.vi" "Field Size"(w479) -> ()
            n239 = local read "Current X (um)"() -> (w488:ext)
            n240 = local read "Current Y (um)"() -> (w487:ext)
            n241 = local read "Current Z (um)"() -> (w485:ext)
          }
          event "Field Number": Value Change {
            n242 = event-data() -> ()  [unwired: 7 out]
            n243 = local read "Field Size"() -> (w514:enum16{"0", "1", "4", "9", "16"})
            n244 = global read "field-raster-globals.vi" "Previous small Z increment"() -> (w504:T3)
            n245 = local read "Current Z (um)"() -> (w505:ext)
            n246 = local write "Current Z 2"(0.0) -> ()
            n247 = Square(x=w514) -> (x^2=w513:u16)
            n248 = Subtract(x=w505, y=w504) -> (x-y=w503:ext)
            n249 = call "field raster.vi"("field size"=w513, "field number"="Field Number") -> ("Plot1"=w510:cluster{dbl[], dbl[]}, "Plot2"=w509:cluster{dbl[], dbl[]}, "current X"=w507:dbl, "current Y"=w508:dbl)  [unwired: 12 in, 2 out]
          }
        }
        n250 = property on="Field Number" class="Slide (strict)"("Maximum"=w38, "Minimum"=w37, "Scale.Minimum"=w37, "Scale.Maximum"=w38) -> ()  [unwired: 2 in, 2 out]
        n251 = global read "field-raster-globals.vi" "Ymax"() -> (w30:dbl)
        n252 = global read "field-raster-globals.vi" "Xmax"() -> (w31:dbl)
        n253 = global read "field-raster-globals.vi" "Zmax"() -> (w32:dbl)
        n254 = In Range and Coerce(upper limit=w30, x=w62, lower limit=w63) -> (coerced(x)=w45:ext, In Range?=w58:bool)
        "Current Y (um)" <- w45
        n255 = In Range and Coerce(upper limit=w31, x=w61, lower limit=w63) -> (coerced(x)=w44:ext, In Range?=w56:bool)
        "Current X (um)" <- w44
        n256 = In Range and Coerce(upper limit=w32, x=w60, lower limit=w63) -> (coerced(x)=w40:ext, In Range?=w54:bool)
        "Current Z (um)" <- w40
        n257 = local write "Current Z"(w40) -> ()
        n258 = call "Nano-drive-usb-SubVI.vi"("Set this axis?"=w50, "Z (um)"=w40, "Y (um)"=w44, "Numeric"=w49, "X (um)"=w45) -> ()  [unwired: 6 in]
        n259 = Not(x=w58) -> (.not. x?=→"At limit":bool)
        n260 = Not(x=w56) -> (.not. x?=→"At limit 2":bool)
        n261 = Not(x=w54) -> (.not. x?=→"At limit 3":bool)
        n262 = Initialize Array(w45, 1) -> (w41:ext[])
        n263 = Initialize Array(w44, 1) -> (w42:ext[])
        n264 = Bundle(w42, w41) -> (w36:cluster{ext[], ext[]})  [unwired: 1 out]
        n265 = Build Array(w36, w35, w34) -> (→"Current (X,Y)":cluster{ext[], ext[]}[])
      }
    }
    frame #2 {
      n266 = call "MCL Release Handle.vi"("handle"=w515) -> ()  [unwired: 10 in, 1 out]
      n267 = Unregister For Events(event registration refnum=w518) -> (error out=w519:errorcluster)  [unwired: 1 in]
      n268 = global write "user event out globals - SubVI.vi" "user event out"(refnum<k0> refnum) -> ()
      n269 = Destroy User Event(user event=w517, error in=w519) -> ()  [unwired: 1 out]
    }
  }
